vi "produce pattern.vi"() -> ()   [LabVIEW 2009]
panel:
  out "Recalculate delay1":bool
  in  "Expected frequency":dbl[unit]
  in  "Expected period":dbl[unit]
  in  "First pulse centered on T/4?":bool
  in  "Delay relative to end of Ch 1?":bool
  out "Ch 2 Digital Waveform Graph":digitalwaveform(graph)
  out "Ch2 output string":string
  out "Ch2width used":dbl[unit]
  out "Ch2delay used":dbl[unit]
  in  "Ch2width":dbl[unit]
  in  "Ch2delay":dbl[unit]
  out "width3 used":dbl[unit]
  out "delay3 used":dbl[unit]
  in  "width3":dbl[unit]
  in  "delay3":dbl[unit]
  out "width2 used":dbl[unit]
  out "delay2 used":dbl[unit]
  out "width1 used":dbl[unit]
  out "delay1 used":dbl[unit]
  in  "width2":dbl[unit]
  in  "delay2":dbl[unit]
  out "time per bit":dbl[unit]
  in  "width1":dbl[unit]
  in  "delay1":dbl[unit]
  out "Ch 1 Digital Waveform Graph":digitalwaveform(graph)
  out "Ch1 output string":string
  in  "Go":bool
  in  "stop":bool
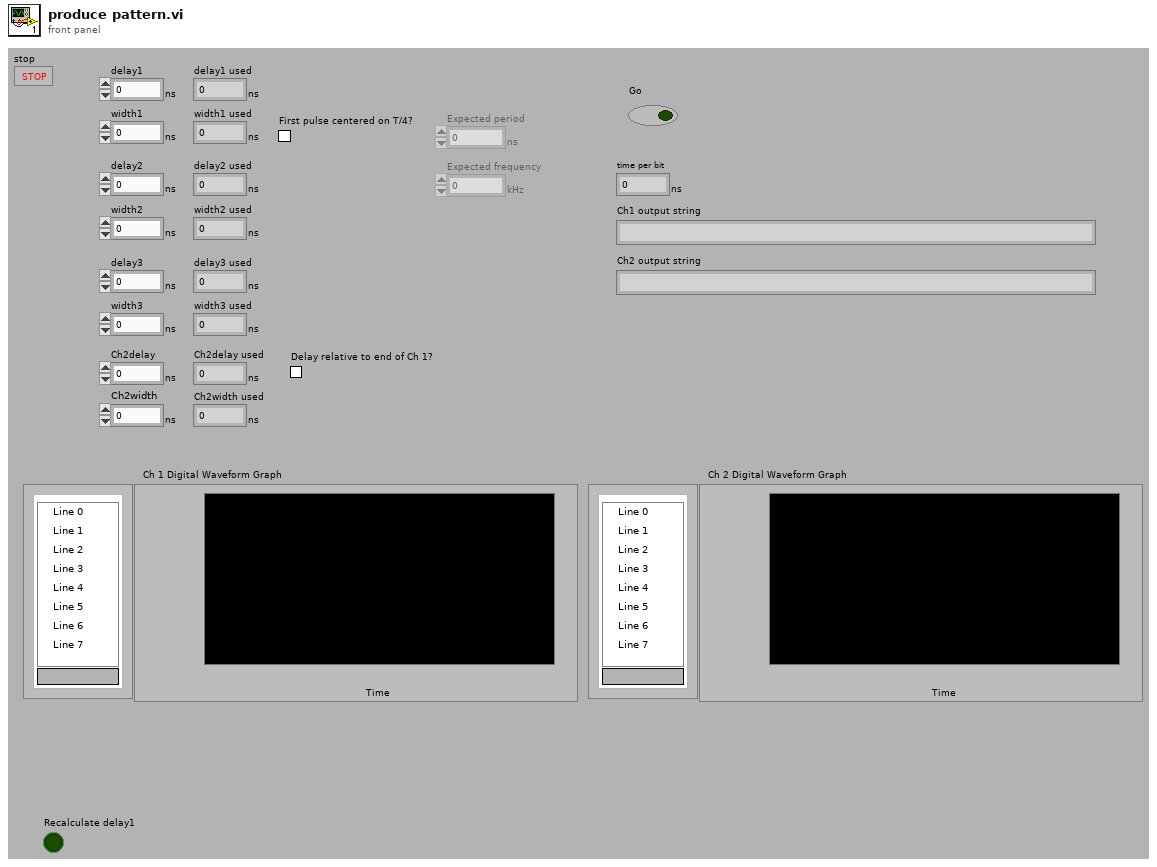
[diagram p1: front panel]
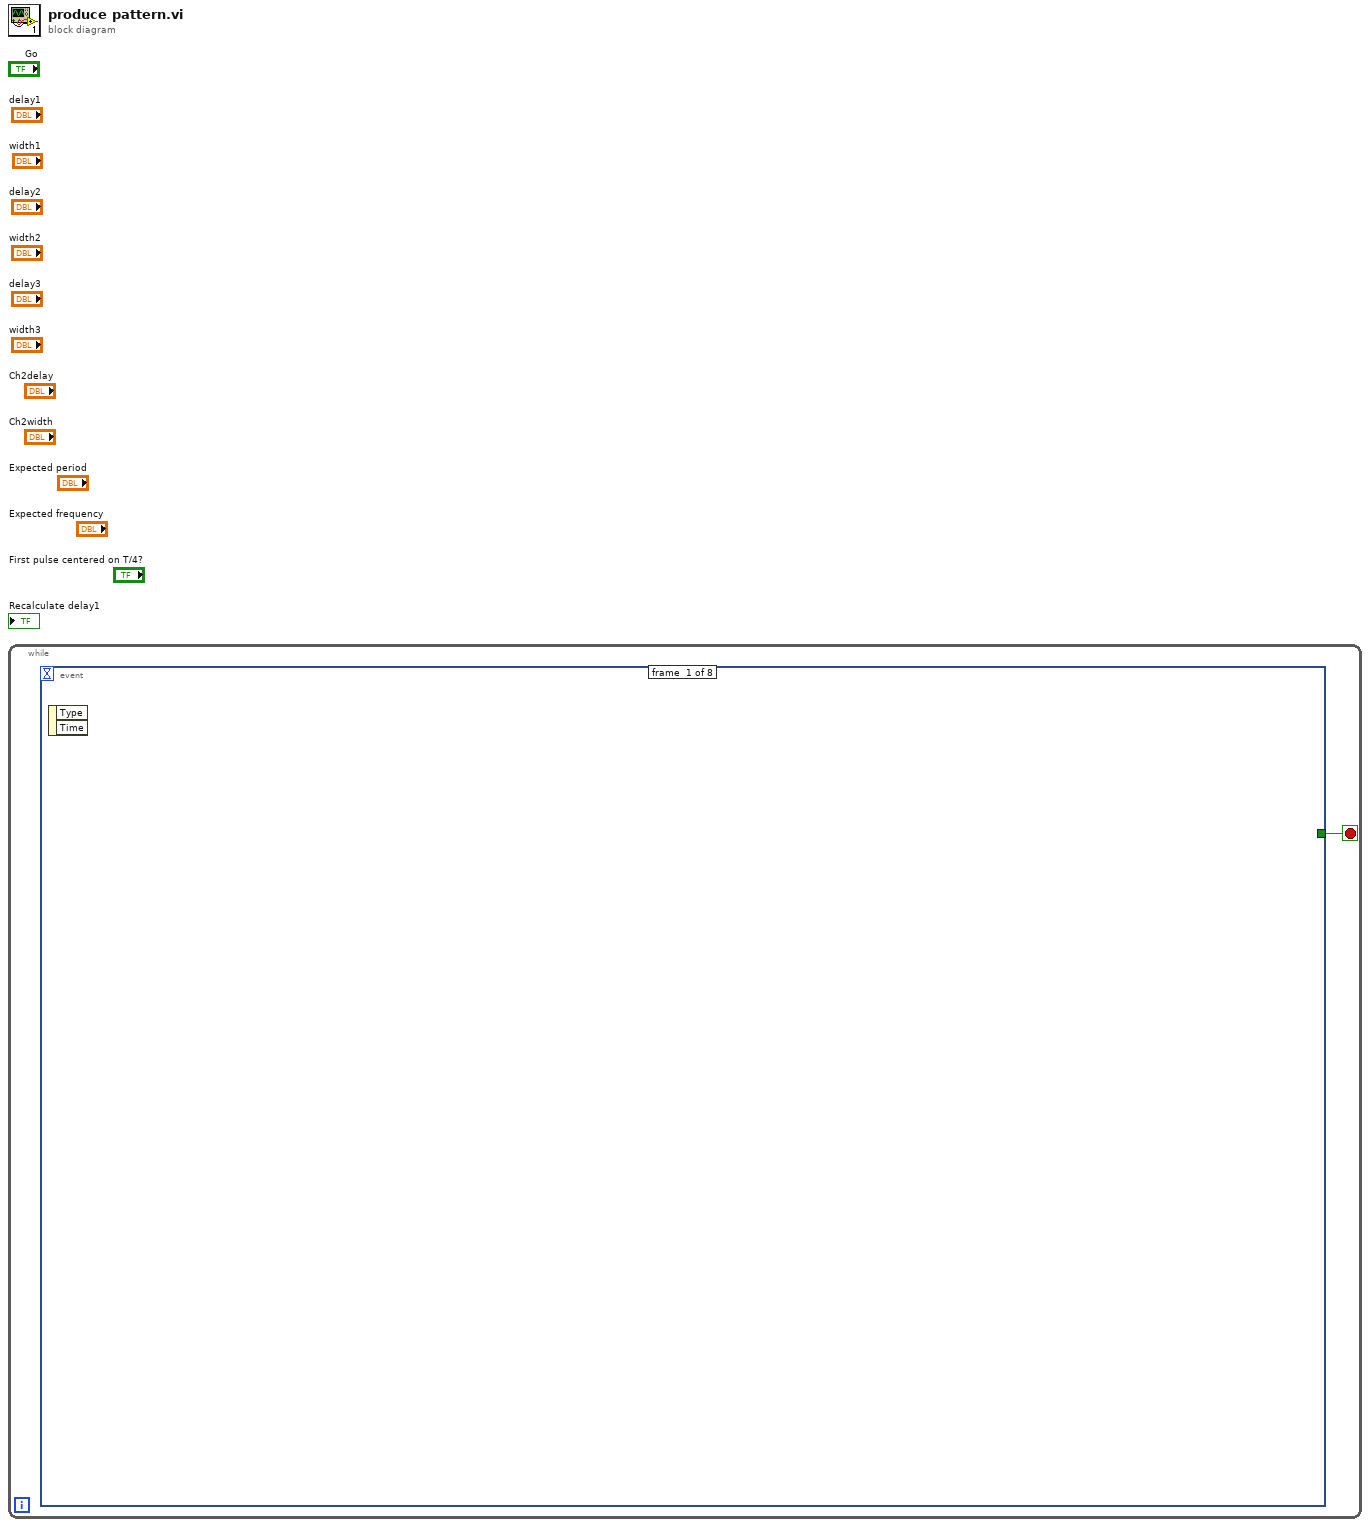
[diagram p0: block diagram]
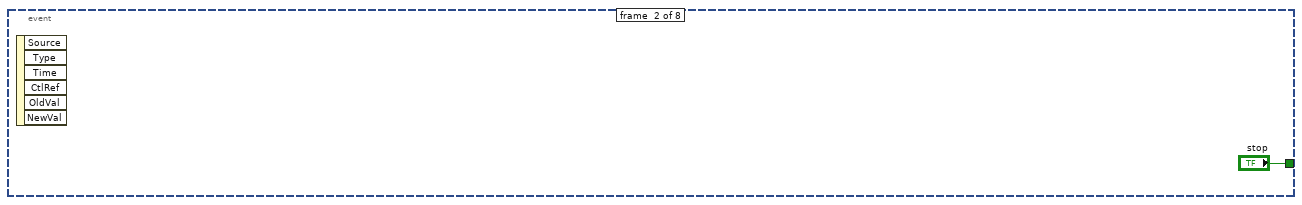
[diagram p2: hidden frame]
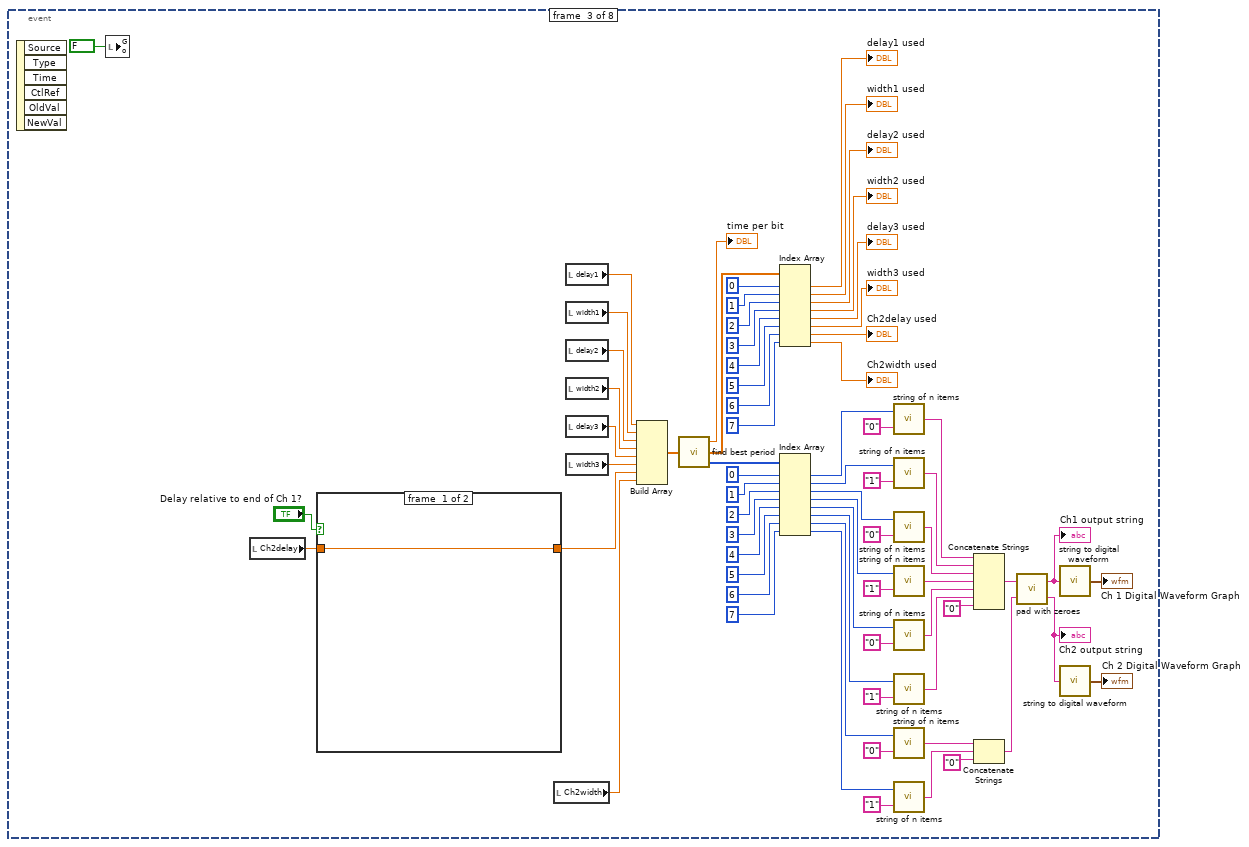
[diagram p3: hidden frame]
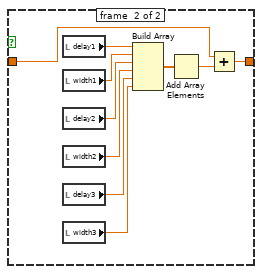
[diagram p4: hidden frame]
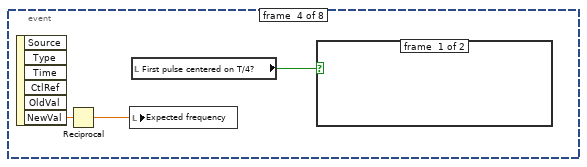
[diagram p5: hidden frame]
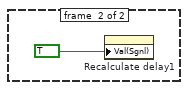
[diagram p6: hidden frame]
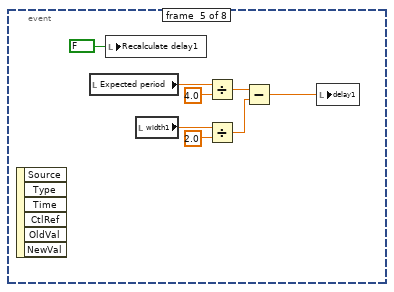
[diagram p7: hidden frame]
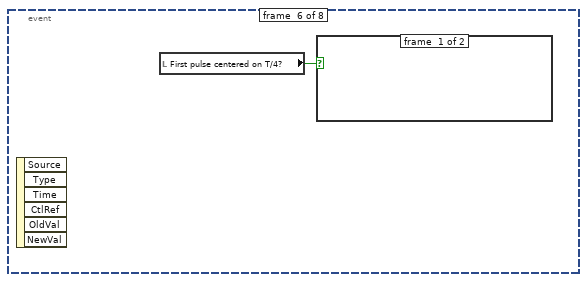
[diagram p8: hidden frame]
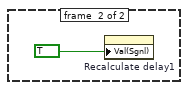
[diagram p9: hidden frame]
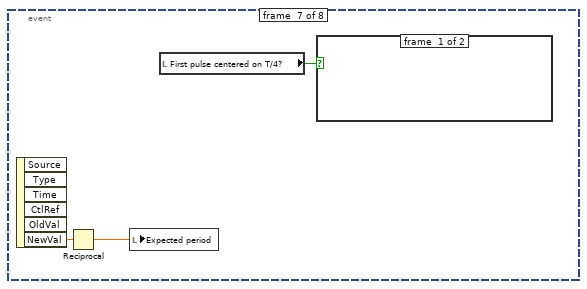
[diagram p10: hidden frame]
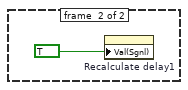
[diagram p11: hidden frame]
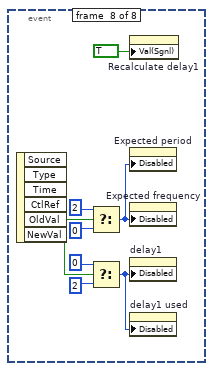
[diagram p12: hidden frame]
diagram:
  n1 = while {
    stop <- w1 stop-if-true
    n2 = event shown="[2] \"Go\": Value Change" {
      selector: _ -> [_ _ _ _ _ _ _ _]
      dyn-events: _ -> [_ _ _ _ _ _ _ _]
      timeout: _ -> [_ _ _ _ _ _ _ _]
      tunnel: [_ "stop" _ _ _ _ _ _] -> w1
      event #0 {
        n3 = event-data() -> ()  [unwired: 3 out]
      }
      event #1 {
        n4 = event-data() -> ()  [unwired: 7 out]
      }
      event #2 {
        n5 = event-data() -> ()  [unwired: 7 out]
        n6 = local write "Go"(FALSE ("Go")) -> ()
        n7 = local read "Ch2delay"() -> (w46:dbl[unit])
        n8 = case shown="True" "Delay relative to end of Ch 1?" {
          tunnel: w46 -> [w74 w84]
          tunnel: [w74 w83] -> w48
          frame #0 {
          }
          frame #1 {
            n9 = local read "delay1"() -> (w81:dbl[unit])
            n10 = local read "width1"() -> (w80:dbl[unit])
            n11 = local read "delay2"() -> (w79:dbl[unit])
            n12 = local read "width2"() -> (w78:dbl[unit])
            n13 = local read "delay3"() -> (w77:dbl[unit])
            n14 = local read "width3"() -> (w76:dbl[unit])
            n15 = Build Array(w81, w80, w79, w78, w77, w76) -> (w75:dbl[unit][])
            n16 = Add Array Elements(numeric array=w75) -> (sum=w82:dbl[unit])
            n17 = Add(x=w84, y=w82) -> (x+y=w83:dbl[unit])
          }
        }
        n18 = local read "Ch2width"() -> (w45:dbl[unit])
        n19 = local read "delay1"() -> (w39:dbl[unit])
        n20 = local read "width1"() -> (w40:dbl[unit])
        n21 = local read "delay2"() -> (w41:dbl[unit])
        n22 = local read "width2"() -> (w42:dbl[unit])
        n23 = local read "delay3"() -> (w43:dbl[unit])
        n24 = local read "width3"() -> (w44:dbl[unit])
        n25 = Build Array(w39, w40, w41, w42, w43, w44, w48, w45) -> (w47:dbl[unit][])
        n26 = call "find best period.vi"("Array of 8 desired times (6 and 2)"=w47) -> ("best period"=→"time per bit":dbl[unit], "Array of 8 actual times (6 and 2)"=w29:dbl[unit][], "Array of 8 \"period-units\" (6 and 2)"=w12:i32[])
        n27 = Index Array(array=w29, index #1=0 ("index"), index #2=1 ("index"), index #3=2 ("index"), index #4=3 ("index"), index #5=4 ("index"), index #6=5 ("index"), index #7=6 ("index"), index #8=7 ("index")) -> (element #1=→"delay1 used":dbl[unit], element #2=→"width1 used":dbl[unit], element #3=→"delay2 used":dbl[unit], element #4=→"width2 used":dbl[unit], element #5=→"delay3 used":dbl[unit], element #6=→"width3 used":dbl[unit], element #7=→"Ch2delay used":dbl[unit], element #8=→"Ch2width used":dbl[unit])
        n28 = Index Array(array=w12, index #1=0 ("index"), index #2=1 ("index"), index #3=2 ("index"), index #4=3 ("index"), index #5=4 ("index"), index #6=5 ("index"), index #7=6 ("index"), index #8=7 ("index")) -> (element #1=w5:i32, element #2=w6:i32, element #3=w7:i32, element #4=w8:i32, element #5=w4:i32, element #6=w3:i32, element #7=w11:i32, element #8=w10:i32)
        n29 = call "string of n items.vi"("string"="0", "Numeric"=w5) -> ("String"=w71:string)
        n30 = call "string of n items.vi"("string"="1", "Numeric"=w6) -> ("String"=w68:string)
        n31 = call "string of n items.vi"("string"="0", "Numeric"=w7) -> ("String"=w65:string)
        n32 = call "string of n items.vi"("string"="1", "Numeric"=w8) -> ("String"=w64:string)
        n33 = call "string of n items.vi"("string"="0", "Numeric"=w4) -> ("String"=w60:string)
        n34 = call "string of n items.vi"("string"="1", "Numeric"=w3) -> ("String"=w59:string)
        n35 = call "string of n items.vi"("string"="0", "Numeric"=w11) -> ("String"=w55:string)
        n36 = call "string of n items.vi"("string"="1", "Numeric"=w10) -> ("String"=w54:string)
        n37 = Concatenate Strings(w71, w68, w65, w64, w60, w59, "0" ("string")) -> (w52:string)
        n38 = Concatenate Strings(w55, w54, "0" ("string")) -> (w51:string)
        n39 = call "pad with zeroes.vi"("String 2 input"=w51, "String 1 input"=w52) -> ("String 2 output"=w50:string, "String 1 output"=w9:string)
        "Ch1 output string" <- w9
        "Ch2 output string" <- w50
        n40 = call "string to digital waveform.vi"("String"=w9) -> ("digital waveform"=→"Ch 1 Digital Waveform Graph":digitalwaveform)
        n41 = call "string to digital waveform.vi"("String"=w50) -> ("digital waveform"=→"Ch 2 Digital Waveform Graph":digitalwaveform)
      }
      event #3 {
        n42 = event-data() -> ("NewVal"=w85:dbl[unit])  [unwired: 6 out]
        n43 = Reciprocal(x=w85) -> (1/x=w87:dbl[unit])
        n44 = local write "Expected frequency"(w87) -> ()
        n45 = local read "First pulse centered on T/4?"() -> (w86:bool)
        n46 = case shown="True" w86 {
          frame #0 {
          }
          frame #1 {
            n47 = property on="Recalculate delay1" class="Bool (strict)"("Val(Sgnl)"=TRUE) -> ()  [unwired: 2 in, 2 out]
          }
        }
      }
      event #4 {
        n48 = event-data() -> ()  [unwired: 7 out]
        n49 = local read "Expected period"() -> (w96:dbl[unit])
        n50 = local write "Recalculate delay1"(FALSE) -> ()
        n51 = local read "width1"() -> (w92:dbl[unit])
        n52 = Divide(x=w96, y=4.0) -> (x/y=w93:dbl[unit])
        n53 = Divide(x=w92, y=2.0) -> (x/y=w90:dbl[unit])
        n54 = Subtract(x=w93, y=w90) -> (x-y=w89:dbl[unit])
        n55 = local write "delay1"(w89) -> ()
      }
      event #5 {
        n56 = event-data() -> ()  [unwired: 7 out]
        n57 = local read "First pulse centered on T/4?"() -> (w97:bool)
        n58 = case shown="True" w97 {
          frame #0 {
          }
          frame #1 {
            n59 = property on="Recalculate delay1" class="Bool (strict)"("Val(Sgnl)"=TRUE ("Value (Signaling)")) -> ()  [unwired: 2 in, 2 out]
          }
        }
      }
      event #6 {
        n60 = event-data() -> ("NewVal"=w101:dbl[unit])  [unwired: 6 out]
        n61 = Reciprocal(x=w101) -> (1/x=w100:dbl[unit])
        n62 = local write "Expected period"(w100) -> ()
        n63 = local read "First pulse centered on T/4?"() -> (w99:bool)
        n64 = case shown="True" w99 {
          frame #0 {
          }
          frame #1 {
            n65 = property on="Recalculate delay1" class="Bool (strict)"("Val(Sgnl)"=TRUE) -> ()  [unwired: 2 in, 2 out]
          }
        }
      }
      event #7 {
        n66 = event-data() -> ("OldVal"=w104:bool)  [unwired: 6 out]
        n67 = Select(t=2, s=w104, f=0) -> (s? t:f=w110:i32)
        n68 = Select(t=0, s=w104, f=2) -> (s? t:f=w105:i32)
        n69 = property on="Recalculate delay1" class="Bool (strict)"("Val(Sgnl)"=TRUE) -> ()  [unwired: 2 in, 2 out]
        n70 = property on="Expected period" class="DigNum (strict)"("Disabled"=w110) -> ()  [unwired: 2 in, 2 out]
        n71 = property on="Expected frequency" class="DigNum (strict)"("Disabled"=w110) -> ()  [unwired: 2 in, 2 out]
        n72 = property on="delay1" class="DigNum (strict)"("Disabled"=w105) -> ()  [unwired: 2 in, 2 out]
        n73 = property on="delay1 used" class="DigNum (strict)"("Disabled"=w105) -> ()  [unwired: 2 in, 2 out]
      }
    }
  }
